vi "PeriodicTriggerProcess.vi"(9 "ID":u32, 10 "time (ms)":i32, 11 "Triggerable":refnum<class "Triggerable.lvclass">) -> ()   [LabVIEW 2020, in "PeriodicTrigger.lvlib"]
uses:
  PeriodicTrigger.lvlib
  Triggerable_interface/Triggerable.lvclass
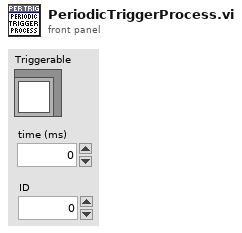
[diagram p1: front panel]
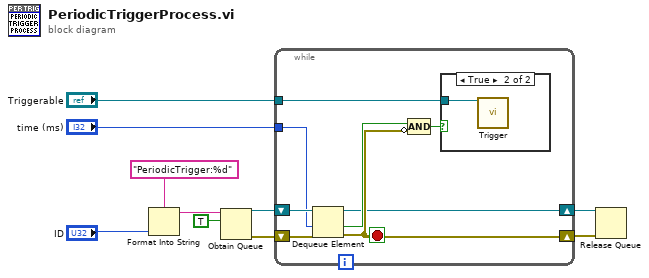
[diagram p0: block diagram]
diagram:
  n1 = Format Into String(format string="PeriodicTrigger:%d", "ID") -> (resulting string=w2:string)  [unwired: 2 in, 1 out]
  n2 = Obtain Queue(name (unnamed)=w2, element data type=TRUE) -> (queue out=w10:refnum<queue>, error out=w9:errorcluster)  [unwired: 3 in, 1 out]
  n3 = while {
    tunnel: "time (ms)" -> [w16]
    tunnel: "Triggerable" -> [w15]
    shift-right: [w11] -> w4
    shift-left: w10 -> [w18]
    shift-right: [w12] -> w5
    shift-left: w9 -> [w17]
    stop <- w12 stop-if-true
    n4 = Dequeue Element(queue=w18, timeout in ms (-1)=w16, error in (no error)=w17) -> (queue out=w11:refnum<queue>, timed out?=w14:bool, error out=w12:errorcluster)  [unwired: 1 out]
    n5 = Compound Arithmetic op=AND(w14, invert w12) -> (w13:bool)
    n6 = case shown="True" w13 {
      tunnel: w15 -> [_ w19]
      frame False {
      }
      frame True {
        n7 = call-dynamic "Trigger.vi"("object in"=w19) -> ()  [unwired: 9 in, 2 out]
      }
    }
  }
  n8 = Release Queue(queue=w4, error in (no error)=w5) -> ()  [unwired: 1 in, 3 out]
